vi "add_tag.vi"(8 "error in (no error)":errorcluster, 10 "tag":string, 11 "Image in":refnum<class "Image.lvclass">) -> (0 "error out":errorcluster, 3 "Image out":refnum<class "Image.lvclass">)   [LabVIEW 2010, in "Image.lvclass"]
uses:
  Image.lvclass
  Image.lvclass/Image.ctl
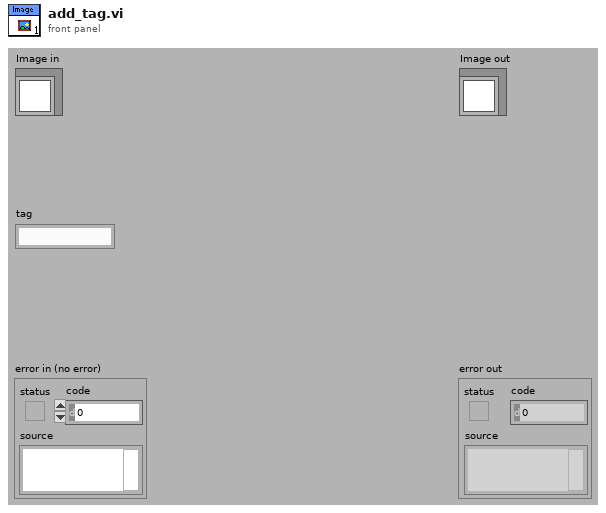
[diagram p1: front panel]
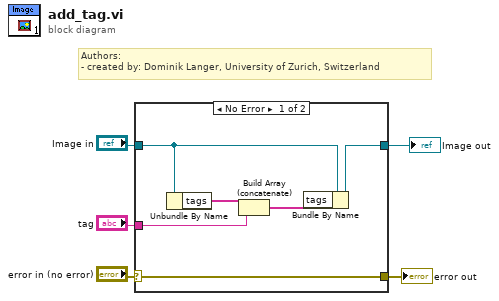
[diagram p0: block diagram]
diagram:
  # "Authors: \n- created by: Dominik Langer, University of Zurich, Switzerland"
  n1 = case shown="No Error" "error in (no error)" {
    selector: "error in (no error)" -> [w11 w13]
    tunnel: [w11 w13] -> w4
    tunnel: [w9 w12] -> w2
    tunnel: "Image in" -> [w10 w12]
    tunnel: "tag" -> [w6 _]
    frame No Error {
      n2 = Unbundle By Name(w10) -> ("tags"=w8:string[])
      n3 = Build Array (concatenate)(w8, w6) -> (w7:string[])
      n4 = Bundle By Name(cluster=w10, "tags"=w7) -> (w9:refnum<class "Image.lvclass">)
    }
    frame Error {
    }
  }
  "error out" <- w4
  "Image out" <- w2
